vi "Test Filter Tests Belonging to Case with Same Suffix.vi"(8 "error in (no error)":errorcluster, 11 "Test Case In":refnum<class "Test Suite Enumeration Test.lvclass">) -> (0 "error out":errorcluster, 3 "Test Case Out":refnum<class "Test Suite Enumeration Test.lvclass">)   [LabVIEW 2020, in "Test Suite Enumeration Test.lvclass"]
uses:
  Test Suite Enumeration Test.lvclass
  C:/Program Files (x86)/National Instruments/LabVIEW 2020/vi.lib/Astemes/LUnit/Core/LUnit Test Case/Test Case.lvclass
  Test Doubles/Debug Test Case Test Double/Case Test Double.lvclass
  Test Doubles/Test Case Test Double/Test Case Test Double.lvclass
  source/Core/Result/Type.ctl
  <vilib>/Astemes/LUnit/Core/LUnit Test Case/Test Case.lvclass/Test Case.ctl
  abc0c33e-1df9-430a-aa1d-b3cbb15f6cba.vi
  <vilib>/Astemes/LUnit/Core/LUnit Test Case/Private/Append Pass Result.vi
  <vilib>/Astemes/LUnit/Core/LUnit Test Case/Private/Append Fail Result.vi
  abc0c33e-1df9-430a-aa1d-b3cbb15f6cba.vi/9c5d11cd-9439-4240-a1ee-d9baace9c924.vi
  <vilib>/Astemes/LUnit/Core/LUnit Test Case/Private/Run In UI.vi
  <vilib>/Utility/error.llb/Clear Errors.vi
  source/LUnit Test Suite.lvclass
  C:/git/astemes-lunit/source/Core/Runnable/Runnable.lvclass
  source/Core/Runnable/Runnable.lvclass
  source/Core/Result/Result.lvlib
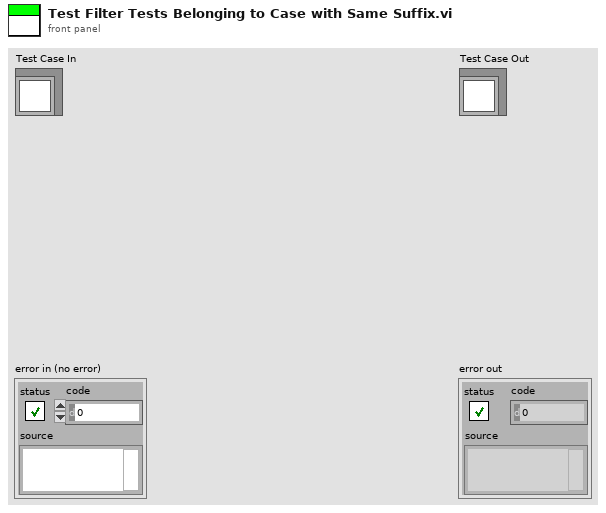
[diagram p1: front panel]
types:
  T1 = typedef "Result.lvlib/Result.ctl" = cluster{"Name":string, "Description":string, "Status":T2, "Result Type":T3, "Execution Time":dbl, "Data":cluster{"Expected":variant, "Actual":variant, "Delta":variant}}
  T2 = typedef "Result.lvlib/Status.ctl" = enum16{"", "Passed", "Failed", "Error", "Skipped", "Setup Error", "Broken", "Teardown Error"}
  T3 = typedef "Result.lvlib/Type.ctl" = enum16{"Test Case", "Test Suite", "Test Run", "Pass", "Fail", "Skip", "Pass if", "Fail if", "Pass if Error", "Fail if Error", "Pass if Equal", "Fail if Equal"}
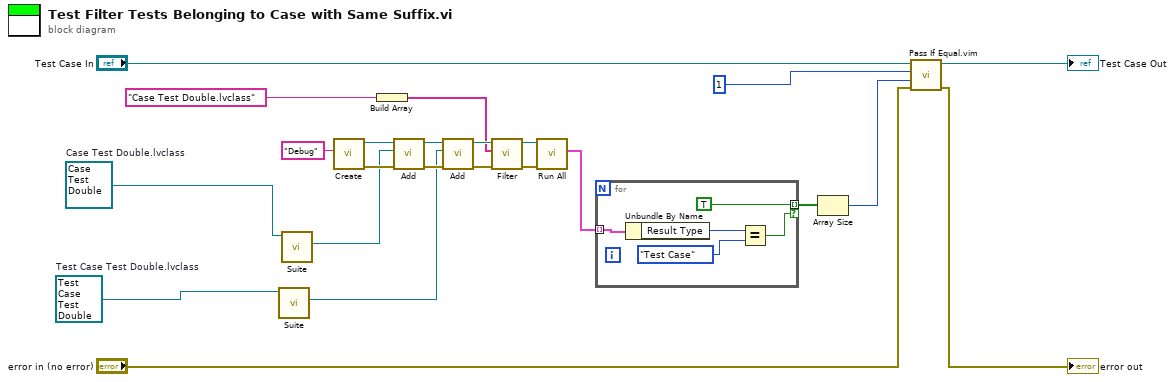
[diagram p0: block diagram]
diagram:
  w14 = refnum<class "Test Case Test Double.lvclass"> refnum  # Test Case Test Double.lvclass
  w19 = refnum<class "Case Test Double.lvclass"> refnum  # Case Test Double.lvclass
  n1 = call-dynamic "Suite.vi"("LUnit Test Case In"=w14) -> ("LUnit Test Suite Out"=w12:refnum<class "LUnit Test Suite.lvclass">)  [unwired: 8 in, 2 out]
  n2 = call-dynamic "Suite.vi"("LUnit Test Case In"=w19) -> ("LUnit Test Suite Out"=w13:refnum<class "LUnit Test Suite.lvclass">)  [unwired: 8 in, 2 out]
  n3 = call "Create.vi"("Suite Name"="Debug") -> ("error out"=w17:errorcluster, "LUnit Test Suite Out"=w18:refnum<class "LUnit Test Suite.lvclass">)  [unwired: 9 in]
  n4 = Build Array("Case Test Double.lvclass") -> (w8:string[])
  n5 = call "Add.vi"("error in (no error)"=w17, "Runnable"=w13, "LUnit Test Suite In"=w18) -> ("error out"=w15:errorcluster, "LUnit Test Suite Out"=w16:refnum<class "LUnit Test Suite.lvclass">)  [unwired: 7 in]
  n6 = call "Add.vi"("error in (no error)"=w15, "Runnable"=w12, "LUnit Test Suite In"=w16) -> ("error out"=w10:errorcluster, "LUnit Test Suite Out"=w11:refnum<class "LUnit Test Suite.lvclass">)  [unwired: 7 in]
  n7 = call "Filter.vi"("error in (no error)"=w10, "Selected Runnables"=w8, "LUnit Test Suite In"=w11) -> ("error out"=w6:errorcluster, "LUnit Test Suite Out"=w7:refnum<class "LUnit Test Suite.lvclass">)  [unwired: 7 in]
  n8 = call "Run All.vi"("error in (no error)"=w6, "Runnable In"=w7) -> ("Results"=w3:T1[])  [unwired: 8 in, 1 out]
  n9 = for {
    tunnel: w3 -> [w28] mode=indexing
    tunnel: [TRUE] -> w2 mode=indexing if=w24
    n10 = Unbundle By Name(w28) -> ("Result Type"=w27:T3)
    n11 = Equal?(x=w27, y=Type."Test Case" ("Result Type")) -> (x = y?=w24:bool)
  }
  n12 = Array Size(array=w2) -> (size(s)=w1:i32)
  n13 = call "Pass If Equal.vim"("error in (no error)"="error in (no error)", "Actual"=w1, "Expected"=1 ("size(s)"), "LUnit Test Case In"="Test Case In") -> ("error out"=→"error out":errorcluster, "LUnit Test Case Out"=→"Test Case Out":refnum<class "Test Suite Enumeration Test.lvclass">)  [unwired: 6 in]
